vi "Set Item Symbol.vi"(8 "Symbol":i32, 10 "Item":string, 11 "Tree in":refnum<class "Tree.lvclass">) -> (3 "Tree out":refnum<class "Tree.lvclass">)   [LabVIEW 2024, in "Tree.lvclass"]
uses:
  Tree.lvclass
  Tree.lvclass/Tree.ctl
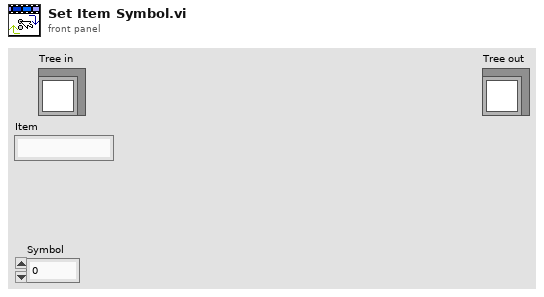
[diagram p1: front panel]
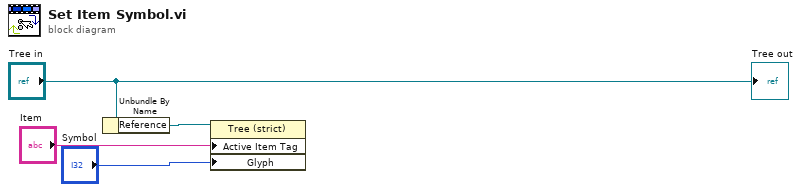
[diagram p0: block diagram]
diagram:
  n1 = Unbundle By Name("Tree in") -> ("Reference"=w3:refnum<vi>)
  n2 = property class="Tree (strict)"(reference=w3, "Active Item Tag"="Item", "Glyph"="Symbol") -> ()  [unwired: 1 in, 2 out]
  "Tree out" <- "Tree in"
